vi "Source V1 and V2.vi"(7 "Slew rate":dbl=5.0, 8 "error in":errorcluster, 9 "V2":dbl, 10 "V1":dbl, 11 "VISA in":refnum<visa-resource-name>) -> (0 "error out":errorcluster, 3 "VISA out":refnum<visa-resource-name>)   [LabVIEW 2016, in "RP100.lvclass"]
uses:
  RP100.lvclass
panel:
  out "out1":string
  out "out2":string
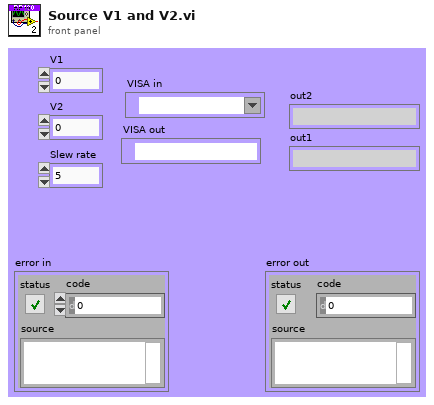
[diagram p1: front panel]
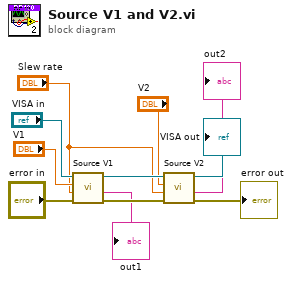
[diagram p0: block diagram]
diagram:
  n1 = call "Source V1.vi"("error in"="error in", "V1 rate"="Slew rate", "V1"="V1", "VISA in"="VISA in") -> ("error out"=w10:errorcluster, "read buffer"=→"out1":string, "VISA out"=w11:refnum<visa-resource-name>)  [unwired: 4 in, 1 out]
  n2 = call "Source V2.vi"("error in"=w10, "V2 rate"="Slew rate", "V2"="V2", "VISA in"=w11) -> ("error out"=→"error out":errorcluster, "read buffer"=→"out2":string, "VISA out"=→"VISA out":refnum<visa-resource-name>)  [unwired: 4 in, 1 out]
